vi "#Function_WaitingTime_LabviewProgram.vi"(8 "error in":errorcluster, 9 "Time":u32) -> (0 "error out":errorcluster, 1 "Boolean":bool=TRUE)   [LabVIEW 2020]
doc: "The function is to wait time (in seconds). It accepts U32."
uses:
  #typedef_Timeenum.ctl
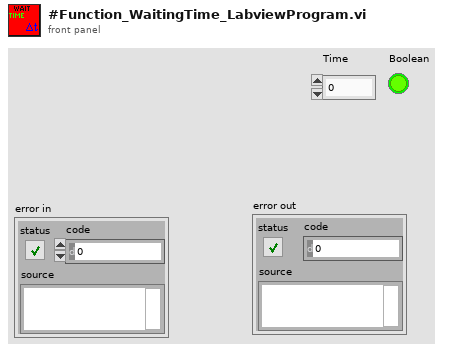
[diagram p1: front panel]
types:
  T1 = typedef "#typedef_Timeenum.ctl" = enum16{"Reset", "Time elapsing"}
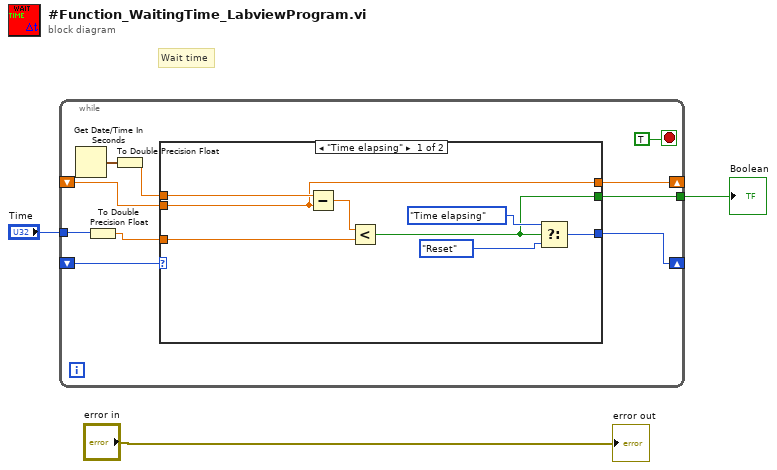
[diagram p0: block diagram]
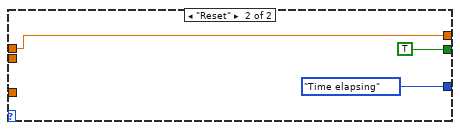
[diagram p2: hidden frame]
diagram:
  # "Wait time"
  n1 = while {
    tunnel: "Time" -> [w10]
    shift-right: [w8] -> _
    shift-left: _ -> [w13]
    tunnel: [w7] -> w1
    shift-right: [w5] -> _
    shift-left: _ -> [w6]
    stop <- TRUE stop-if-true
    n2 = Get Date/Time In Seconds() -> (seconds since 1Jan1904=w12:timestamp)
    n3 = To Double Precision Float(number=w10) -> (double precision float=w9:dbl)
    n4 = To Double Precision Float(number=w12) -> (double precision float=w11:dbl)
    n5 = case shown="\"Time elapsing\"" w13 {
      tunnel: w11 -> [w21 w24]
      tunnel: w9 -> [w20 _]
      tunnel: [w17 #typedef_Timeenum."Time elapsing"] -> w8
      tunnel: [w16 TRUE] -> w7
      tunnel: w6 -> [w15 _]
      tunnel: [w15 w24] -> w5
      frame "Time elapsing" {
        n6 = Subtract(x=w21, y=w15) -> (x-y=w14:dbl)
        n7 = Less?(x=w14, y=w20) -> (x < y?=w16:bool)
        n8 = Select(t=#typedef_Timeenum."Time elapsing", s=w16, f=#typedef_Timeenum."Reset") -> (s? t:f=w17:T1)
      }
      frame "Reset" {
      }
    }
  }
  "Boolean" <- w1
  "error out" <- "error in"
